vi "Test.vi"() -> ()   [LabVIEW 2023]
uses:
  Proto_client/Proto_client.lvlib
  Proto_client/RPC Messages/grpcservice_AkipResponse.ctl
panel:
  out "error out":errorcluster
  out "Response Data":T1
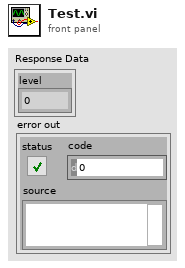
[diagram p1: front panel]
types:
  T1 = typedef "Proto_client.lvlib/grpcservice_AkipResponse.ctl" = cluster{"level":sgl}
  T2 = typedef "grpc-lvsupport-release.lvlib/grpcId.ctl" = u64
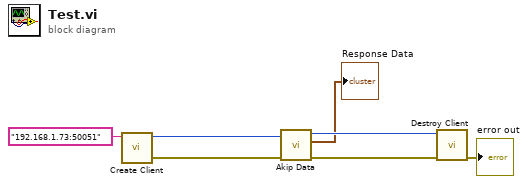
[diagram p0: block diagram]
diagram:
  n1 = call "Create Client.vi"("address"="192.168.1.73:50051") -> ("error out"=w6:errorcluster, "gRPC ID Out"=w7:T2)  [unwired: 9 in]
  n2 = call "Akip Data.vi"("error in"=w6, "gRPC ID"=w7) -> ("error out"=w4:errorcluster, "Response Data"=→"Response Data":T1, "gRPC ID out"=w3:T2)  [unwired: 7 in]
  n3 = call "Destroy Client.vi"("error in"=w4, "gRPC ID"=w3) -> ("error out"=→"error out":errorcluster)  [unwired: 9 in]
